vi "PersonnelFGV.vi"(7 "Actions":T1=enum."Read Personnel", 8 "error in (no error)":errorcluster, 9 "Data In":string, 10 "PUID":string) -> (0 "error out":errorcluster, 1 "Data Out":string)   [LabVIEW 2015]
uses:
  TypeDef/PersonnelActions.ctl
  TypeDef/PersonnelState.ctl
  LVClasses/Personnel/Personnel.lvclass
  LVClasses/Personnel/PersonnelType.ctl
  LVClasses/Personnel/Personnel.lvclass/Personnel.ctl
  LVClasses/Personnel/Read Name.vi
  LVClasses/Personnel/Read Role.vi
  LVClasses/Personnel/Read UniqueID.vi
  LVClasses/Personnel/Read Requests.vi
  LVClasses/Personnel/Write Requests.vi
  LVClasses/Personnel/Write Name.vi
  LVClasses/Personnel/Write Role.vi
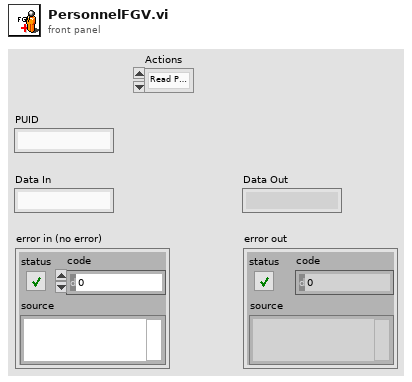
[diagram p1: front panel]
types:
  T1 = typedef "PersonnelActions.ctl" = enum16{"Init", "Read Personnel", "Add Personnel", "Remove Personnel", "Read Name", "Write Name", "Read Role", "Write Role", "Read Requests", "Add Requests", "Remove Requests", "Read PUIDs"}
  T2 = typedef "PersonnelState.ctl" = cluster{"Personnel":refnum<class "Personnel.lvclass">[]}
  T3 = typedef "Personnel.lvclass/PersonnelType.ctl" = enum16{"Nurse", "Doctor", "Cleanning", "Admin"}
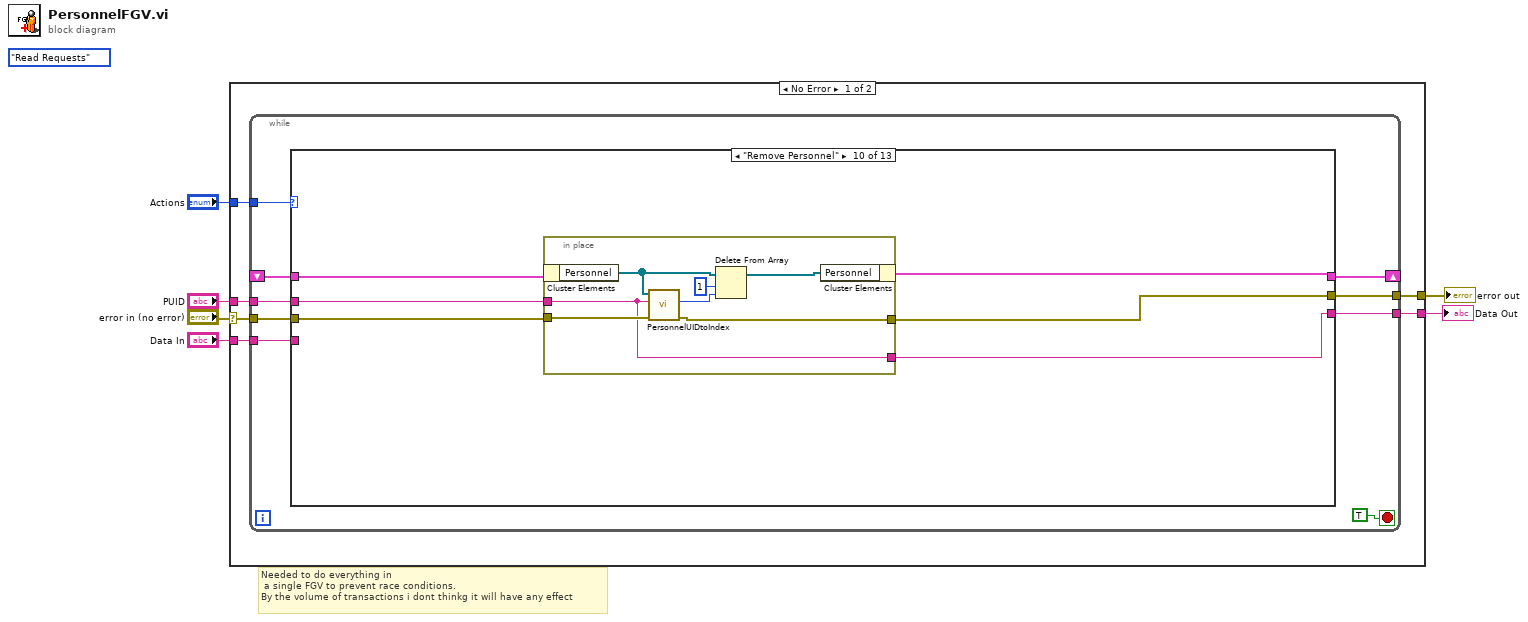
[diagram p0: block diagram]
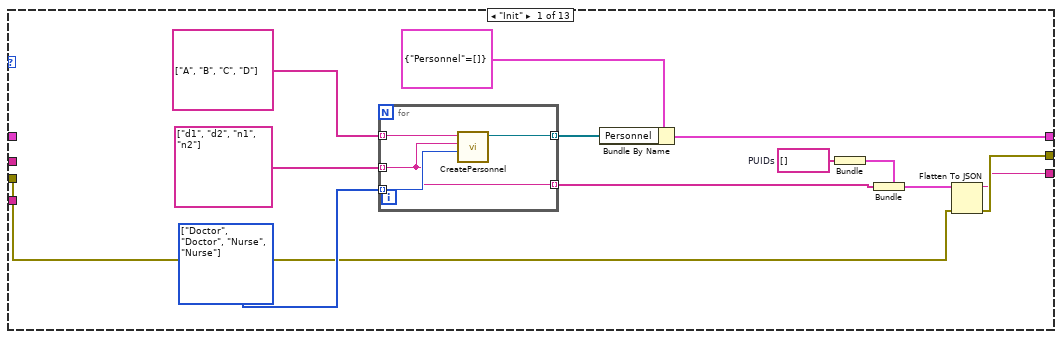
[diagram p2: hidden frame]
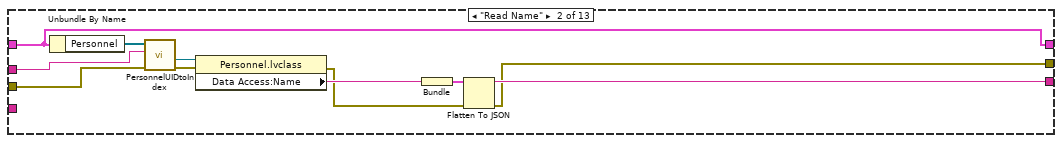
[diagram p3: hidden frame]
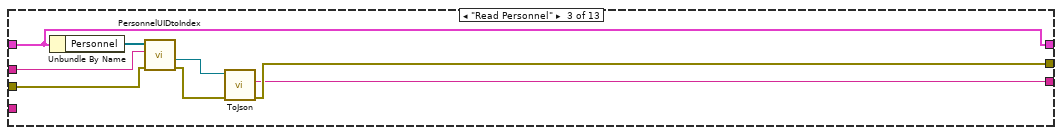
[diagram p4: hidden frame]
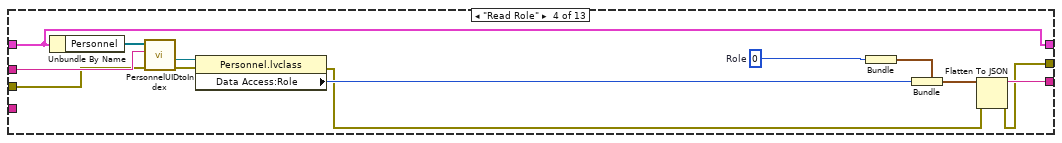
[diagram p5: hidden frame]
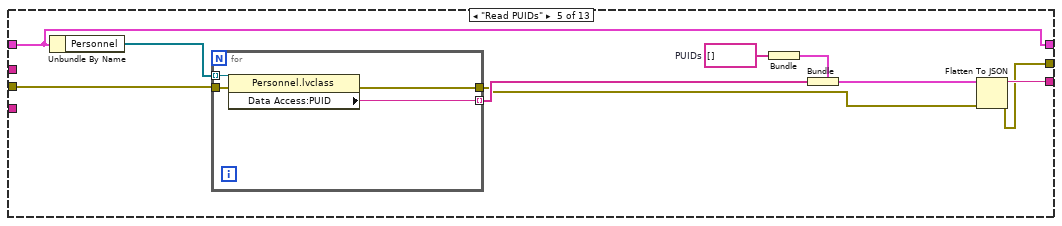
[diagram p6: hidden frame]
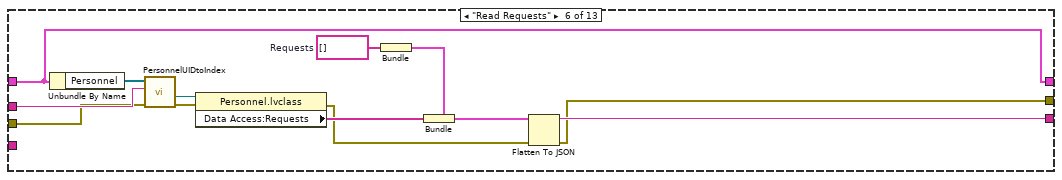
[diagram p7: hidden frame]
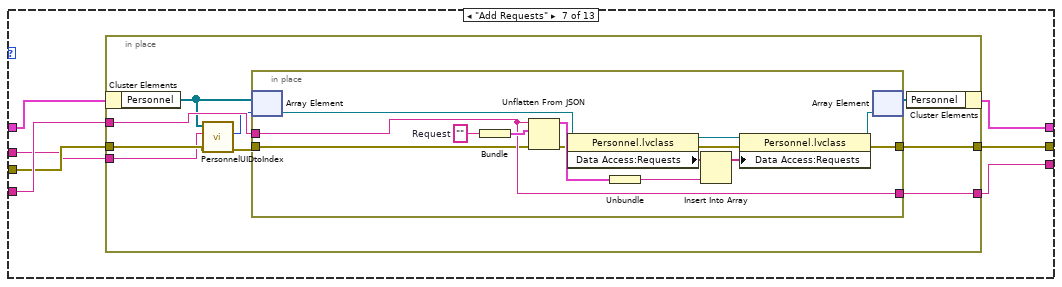
[diagram p8: hidden frame]
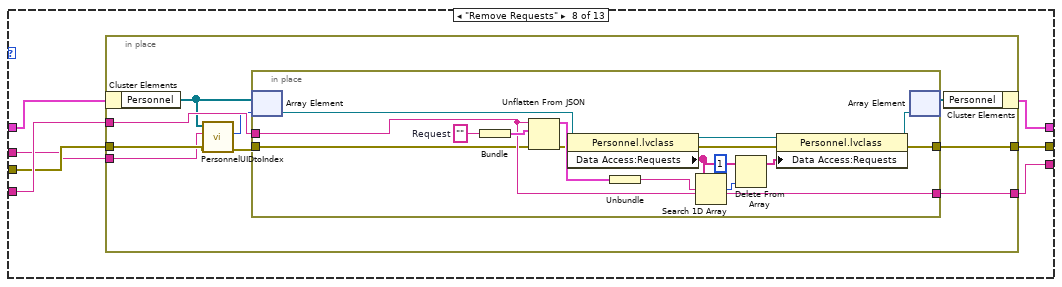
[diagram p9: hidden frame]
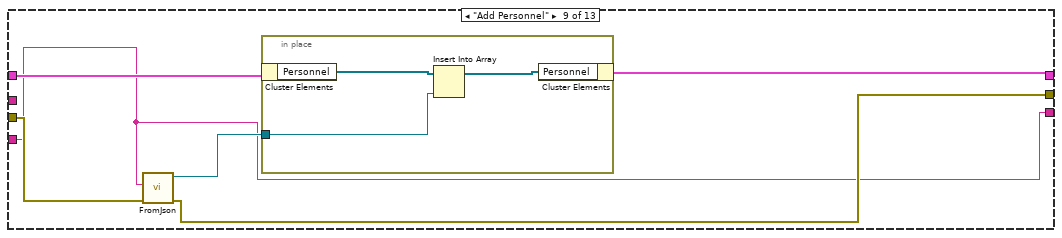
[diagram p10: hidden frame]
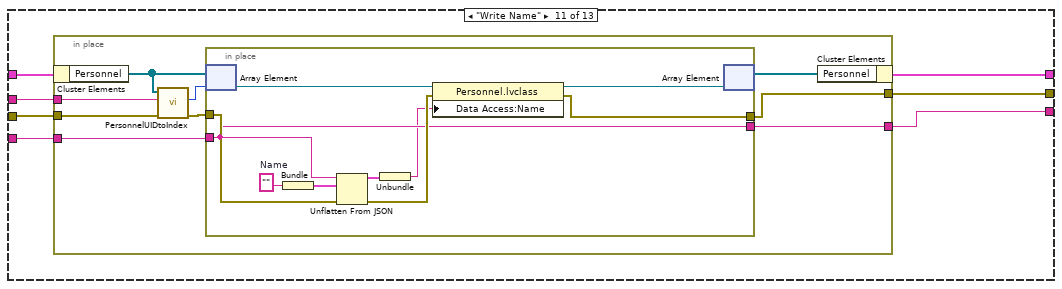
[diagram p11: hidden frame]
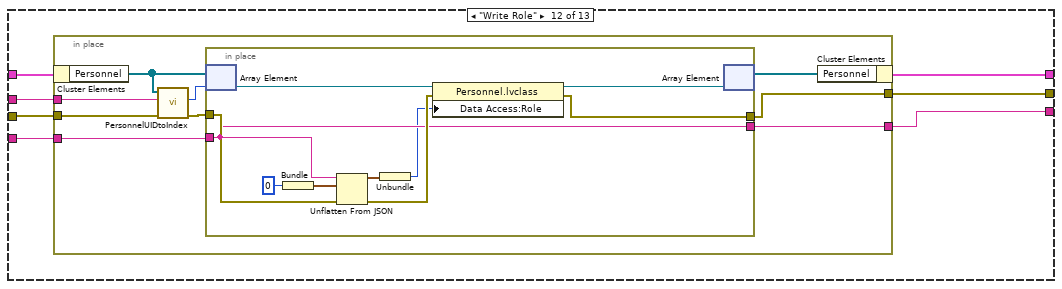
[diagram p12: hidden frame]
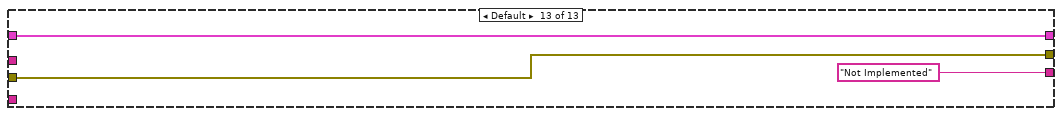
[diagram p13: hidden frame]
diagram:
  (unwired) PersonnelActions."Read Requests" ("Actions")
  # "Needed to do everything in\n a single FGV to prevent race conditions. \nBy the volume of transactions i dont thinkg it will have any effect"
  n1 = case shown="No Error" "error in (no error)" {
    selector: "error in (no error)" -> [w8 w237]
    tunnel: "Actions" -> [w12 _]
    tunnel: "PUID" -> [w11 _]
    tunnel: [w10 _] -> w4
    tunnel: "Data In" -> [w9 _]
    tunnel: [w7 w237] -> w1
    frame No Error {
      n2 = while {
        shift-right: [w19] -> _
        shift-left: _ -> [w18]
        tunnel: w12 -> [w20]
        tunnel: w11 -> [w17]
        tunnel: [w16] -> w10
        tunnel: w9 -> [w15]
        tunnel: w8 -> [w14]
        tunnel: [w13] -> w7
        stop <- TRUE ("stop") stop-if-true
        n3 = case shown="\"Remove Personnel\"" w20 {
          tunnel: [w34 w49 w57 w70 w80 w97 w99 w129 w161 w173 w187 w213 w236] -> w19
          tunnel: w18 -> [_ w49 w57 w70 w80 w97 w104 w134 w165 w174 w188 w214 w236]
          tunnel: w17 -> [_ w47 w55 w68 _ w95 w100 w130 _ w170 w184 w210 _]
          tunnel: [w22 w43 w50 w64 w79 w93 w98 w128 w160 w169 w182 w208 "Not Implemented" ("JSON string")] -> w16
          tunnel: w15 -> [_ _ _ _ _ _ w103 w133 w160 _ w183 w209 _]
          tunnel: w14 -> [w25 w42 w54 w61 w72 w88 w102 w132 w164 w172 w186 w212 w234]
          tunnel: [w26 w39 w51 w58 w78 w85 w101 w131 w163 w171 w185 w211 w234] -> w13
          frame "Init" {
            w27 = string[] []  # PUIDs
            w31 = T3[] [enum."Doctor", enum."Doctor", enum."Nurse", enum."Nurse"] items=["Nurse", "Doctor", "Cleanning", "Admin"]
            n4 = for {
              tunnel: [w38] -> w32 mode=indexing
              tunnel: w31 -> [w37] mode=indexing
              tunnel: string[] ["d1", "d2", "n1", "n2"] -> [w35] mode=indexing
              tunnel: string[] ["A", "B", "C", "D"] -> [w36] mode=indexing
              tunnel: [w35] -> w23 mode=indexing
              n5 = call "CreatePersonnel.vi"("Role"=w37, "UniqueID"=w35, "Name"=w36) -> ("output cluster"=w38:refnum<class "Personnel.lvclass">)  [unwired: 7 in, 1 out]
            }
            n6 = Bundle By Name(cluster=T2 {"Personnel"=[]}, "Personnel"=w32) -> (w34:T2)
            n7 = Bundle("PUIDs"=w27) -> (w28:cluster{"PUIDs":string[]})  [unwired: 1 in]
            n8 = Bundle(cluster=w28, "PUIDs"=w23) -> (w24:cluster{"PUIDs":string[]})
            n9 = Flatten To JSON(anything=w24, error in (no error)=w25) -> (JSON string=w22:string, 11:w26:errorcluster)  [unwired: 1 in]
          }
          frame "Read Name" {
            n10 = Unbundle By Name(w49) -> ("Personnel"=w48:refnum<class "Personnel.lvclass">[])
            n11 = call "PersonnelUIDtoIndex.vi"("error in (no error)"=w42, "PUID"=w47, "Personnel in"=w48) -> ("error out"=w41:errorcluster, "Personnel"=w46:refnum<class "Personnel.lvclass">)  [unwired: 5 in, 2 out]
            n12 = property class="Personnel.lvclass"(reference=w46, error in=w41) -> (error out=w40:errorcluster, "Data Access:Name"=w45:string)  [unwired: 1 out]
            n13 = Bundle("Data Access:Name"=w45) -> (w44:cluster{"Data Access:Name":string})  [unwired: 1 in]
            n14 = Flatten To JSON(anything=w44, error in (no error)=w40) -> (JSON string=w43:string, 11:w39:errorcluster)  [unwired: 1 in]
          }
          frame "Read Personnel" {
            n15 = Unbundle By Name(w57) -> ("Personnel"=w56:refnum<class "Personnel.lvclass">[])
            n16 = call "PersonnelUIDtoIndex.vi"("error in (no error)"=w54, "PUID"=w55, "Personnel in"=w56) -> ("error out"=w53:errorcluster, "Personnel"=w52:refnum<class "Personnel.lvclass">)  [unwired: 5 in, 2 out]
            n17 = call "ToJson.vi"("error in (no error)"=w53, "Personnel in"=w52) -> ("error out"=w51:errorcluster, "PersonnelJson"=w50:string)  [unwired: 7 in, 1 out]
          }
          frame "Read Role" {
            w63 = 0  # Role
            n18 = Unbundle By Name(w70) -> ("Personnel"=w69:refnum<class "Personnel.lvclass">[])
            n19 = call "PersonnelUIDtoIndex.vi"("error in (no error)"=w61, "PUID"=w68, "Personnel in"=w69) -> ("error out"=w60:errorcluster, "Personnel"=w67:refnum<class "Personnel.lvclass">)  [unwired: 5 in, 2 out]
            n20 = property class="Personnel.lvclass"(reference=w67, error in=w60) -> (error out=w59:errorcluster, "Data Access:Role"=w66:T3)  [unwired: 1 out]
            n21 = Bundle("Role"=w63) -> (w62:cluster{"Role":i32})  [unwired: 1 in]
            n22 = Bundle(cluster=w62, "Role"=w66) -> (w65:cluster{"Role":i32})
            n23 = Flatten To JSON(anything=w65, error in (no error)=w59) -> (JSON string=w64:string, 11:w58:errorcluster)  [unwired: 1 in]
          }
          frame "Read PUIDs" {
            w75 = string[] []  # PUIDs
            n24 = Unbundle By Name(w80) -> ("Personnel"=w77:refnum<class "Personnel.lvclass">[])
            n25 = for {
              tunnel: w77 -> [w84] mode=indexing
              tunnel: [w83] -> w73 mode=indexing
              tunnel: w72 -> [w82]
              tunnel: [w81] -> w71
              n26 = property class="Personnel.lvclass"(reference=w84, error in=w82) -> (error out=w81:errorcluster, "Data Access:PUID"=w83:string)  [unwired: 1 out]
            }
            n27 = Bundle("PUIDs"=w75) -> (w76:cluster{"PUIDs":string[]})  [unwired: 1 in]
            n28 = Bundle(cluster=w76, "PUIDs"=w73) -> (w74:cluster{"PUIDs":string[]})
            n29 = Flatten To JSON(anything=w74, error in (no error)=w71) -> (JSON string=w79:string, 11:w78:errorcluster)  [unwired: 1 in]
          }
          frame "Read Requests" {
            w91 = string[] []  # Requests
            n30 = Unbundle By Name(w97) -> ("Personnel"=w96:refnum<class "Personnel.lvclass">[])
            n31 = call "PersonnelUIDtoIndex.vi"("error in (no error)"=w88, "PUID"=w95, "Personnel in"=w96) -> ("error out"=w87:errorcluster, "Personnel"=w94:refnum<class "Personnel.lvclass">)  [unwired: 5 in, 2 out]
            n32 = property class="Personnel.lvclass"(reference=w94, error in=w87) -> (error out=w86:errorcluster, "Data Access:Requests"=w90:string[])  [unwired: 1 out]
            n33 = Bundle("Requests"=w91) -> (w92:cluster{"Requests":string[]})  [unwired: 1 in]
            n34 = Bundle(cluster=w92, "Requests"=w90) -> (w89:cluster{"Requests":string[]})
            n35 = Flatten To JSON(anything=w89, error in (no error)=w86) -> (JSON string=w93:string, 11:w85:errorcluster)  [unwired: 1 in]
          }
          frame "Add Requests" {
            n36 = in-place {
              in-place-border: [w111] -> w98
              in-place-border: w102 -> [w106]
              in-place-border: [w112] -> w101
              in-place-border: w103 -> [w110]
              in-place-border: w100 -> [w105]
              n37 = in-place-cluster #1(w104) -> ("Personnel"=w109:refnum<class "Personnel.lvclass">[])
              n38 = call "PersonnelUIDtoIndex.vi"("error in (no error)"=w106, "PUID"=w105, "Personnel in"=w109) -> ("error out"=w107:errorcluster, "Index"=w108:i32)  [unwired: 5 in, 2 out]
              n39 = in-place {
                in-place-border: w107 -> [w121]
                in-place-border: [w127] -> w112
                in-place-border: [w124] -> w111
                in-place-border: w110 -> [w124]
                w120 = ""  # Request
                n40 = in-place-array #2(w109, w108) -> (w122:refnum<class "Personnel.lvclass">)
                n41 = Bundle("Request"=w120) -> (w125:cluster{"Request":string})  [unwired: 1 in]
                n42 = Unflatten From JSON(JSON string=w124, type and defaults=w125, error in (no error)=w121) -> (value=w123:cluster{"Request":string}, error out=w118:errorcluster)  [unwired: 4 in]
                n43 = property class="Personnel.lvclass"(reference=w122, error in=w118) -> (reference out=w119:refnum<class "Personnel.lvclass">, error out=w117:errorcluster, "Data Access:Requests"=w116:string[])
                n44 = Unbundle(w123) -> ("Request"=w114:string)
                n45 = Insert Into Array(array=w116, new element=w114) -> (w115:string[])  [unwired: 1 in]
                n46 = property class="Personnel.lvclass"(reference=w119, error in=w117, "Data Access:Requests"=w115) -> (reference out=w126:refnum<class "Personnel.lvclass">, error out=w127:errorcluster)
                n47 = in-place-array #2(w126) -> (w113:refnum<class "Personnel.lvclass">[])  [unwired: 1 out]
              }
              n48 = in-place-cluster #1("Personnel"=w113) -> (w99:T2)
            }
          }
          frame "Remove Requests" {
            n49 = in-place {
              in-place-border: [w141] -> w128
              in-place-border: w132 -> [w136]
              in-place-border: [w142] -> w131
              in-place-border: w133 -> [w140]
              in-place-border: w130 -> [w135]
              n50 = in-place-cluster #3(w134) -> ("Personnel"=w139:refnum<class "Personnel.lvclass">[])
              n51 = call "PersonnelUIDtoIndex.vi"("error in (no error)"=w136, "PUID"=w135, "Personnel in"=w139) -> ("error out"=w137:errorcluster, "Index"=w138:i32)  [unwired: 5 in, 2 out]
              n52 = in-place {
                in-place-border: w137 -> [w153]
                in-place-border: [w159] -> w142
                in-place-border: [w156] -> w141
                in-place-border: w140 -> [w156]
                w152 = ""  # Request
                n53 = in-place-array #4(w139, w138) -> (w154:refnum<class "Personnel.lvclass">)
                n54 = Bundle("Request"=w152) -> (w157:cluster{"Request":string})  [unwired: 1 in]
                n55 = Unflatten From JSON(JSON string=w156, type and defaults=w157, error in (no error)=w153) -> (value=w155:cluster{"Request":string}, error out=w150:errorcluster)  [unwired: 4 in]
                n56 = property class="Personnel.lvclass"(reference=w154, error in=w150) -> (reference out=w151:refnum<class "Personnel.lvclass">, error out=w149:errorcluster, "Data Access:Requests"=w148:string[])
                n57 = Unbundle(w155) -> ("Request"=w144:string)
                n58 = Search 1D Array(1D array=w148, element=w144) -> (index of element=w146:i32)  [unwired: 1 in]
                n59 = Delete From Array(array=w148, length=1, index=w146) -> (array with subset deleted=w147:string[])  [unwired: 1 out]
                n60 = property class="Personnel.lvclass"(reference=w151, error in=w149, "Data Access:Requests"=w147) -> (reference out=w158:refnum<class "Personnel.lvclass">, error out=w159:errorcluster)
                n61 = in-place-array #4(w158) -> (w143:refnum<class "Personnel.lvclass">[])  [unwired: 1 out]
              }
              n62 = in-place-cluster #3("Personnel"=w143) -> (w129:T2)
            }
          }
          frame "Add Personnel" {
            n63 = call "FromJson.vi"("error in (no error)"=w164, "PersonnelJson"=w160) -> ("error out"=w163:errorcluster, "Personnel out"=w162:refnum<class "Personnel.lvclass">)  [unwired: 8 in]
            n64 = in-place {
              in-place-border: w162 -> [w166]
              n65 = in-place-cluster #5(w165) -> ("Personnel"=w168:refnum<class "Personnel.lvclass">[])
              n66 = Insert Into Array(array=w168, new element=w166) -> (w167:refnum<class "Personnel.lvclass">[])  [unwired: 1 in]
              n67 = in-place-cluster #5("Personnel"=w167) -> (w161:T2)
            }
          }
          frame "Remove Personnel" {
            n68 = in-place {
              in-place-border: w170 -> [w175]
              in-place-border: w172 -> [w180]
              in-place-border: [w176] -> w171
              in-place-border: [w175] -> w169
              n69 = in-place-cluster #6(w174) -> ("Personnel"=w179:refnum<class "Personnel.lvclass">[])
              n70 = call "PersonnelUIDtoIndex.vi"("error in (no error)"=w180, "PUID"=w175, "Personnel in"=w179) -> ("error out"=w176:errorcluster, "Index"=w177:i32)  [unwired: 5 in, 2 out]
              n71 = Delete From Array(array=w179, length=1, index=w177) -> (array with subset deleted=w181:refnum<class "Personnel.lvclass">[])  [unwired: 1 out]
              n72 = in-place-cluster #6("Personnel"=w181) -> (w173:T2)
            }
          }
          frame "Write Name" {
            n73 = in-place {
              in-place-border: w184 -> [w197]
              in-place-border: w186 -> [w196]
              in-place-border: [w190] -> w185
              in-place-border: w183 -> [w192]
              in-place-border: [w189] -> w182
              n74 = in-place-cluster #7(w188) -> ("Personnel"=w195:refnum<class "Personnel.lvclass">[])
              n75 = call "PersonnelUIDtoIndex.vi"("error in (no error)"=w196, "PUID"=w197, "Personnel in"=w195) -> ("error out"=w191:errorcluster, "Index"=w193:i32)  [unwired: 5 in, 2 out]
              n76 = in-place {
                in-place-border: w192 -> [w202]
                in-place-border: w191 -> [w205]
                in-place-border: [w203] -> w190
                in-place-border: [w202] -> w189
                w201 = ""  # Name
                n77 = in-place-array #8(w195, w193) -> (w207:refnum<class "Personnel.lvclass">)
                n78 = Bundle("Name"=w201) -> (w200:cluster{"Name":string})  [unwired: 1 in]
                n79 = Unflatten From JSON(JSON string=w202, type and defaults=w200, error in (no error)=w205) -> (value=w199:cluster{"Name":string}, error out=w204:errorcluster)  [unwired: 4 in]
                n80 = Unbundle(w199) -> ("Name"=w198:string)
                n81 = property class="Personnel.lvclass"(reference=w207, error in=w204, "Data Access:Name"=w198) -> (reference out=w206:refnum<class "Personnel.lvclass">, error out=w203:errorcluster)
                n82 = in-place-array #8(w206) -> (w194:refnum<class "Personnel.lvclass">[])  [unwired: 1 out]
              }
              n83 = in-place-cluster #7("Personnel"=w194) -> (w187:T2)
            }
          }
          frame "Write Role" {
            n84 = in-place {
              in-place-border: w210 -> [w223]
              in-place-border: w212 -> [w222]
              in-place-border: [w216] -> w211
              in-place-border: w209 -> [w218]
              in-place-border: [w215] -> w208
              n85 = in-place-cluster #9(w214) -> ("Personnel"=w221:refnum<class "Personnel.lvclass">[])
              n86 = call "PersonnelUIDtoIndex.vi"("error in (no error)"=w222, "PUID"=w223, "Personnel in"=w221) -> ("error out"=w217:errorcluster, "Index"=w219:i32)  [unwired: 5 in, 2 out]
              n87 = in-place {
                in-place-border: w218 -> [w228]
                in-place-border: w217 -> [w231]
                in-place-border: [w229] -> w216
                in-place-border: [w228] -> w215
                n88 = in-place-array #10(w221, w219) -> (w233:refnum<class "Personnel.lvclass">)
                n89 = Bundle("Role"=0) -> (w227:cluster{"Role":i32})  [unwired: 1 in]
                n90 = Unflatten From JSON(JSON string=w228, type and defaults=w227, error in (no error)=w231) -> (value=w226:cluster{"Role":i32}, error out=w230:errorcluster)  [unwired: 4 in]
                n91 = Unbundle(w226) -> ("Role"=w225:i32)
                n92 = property class="Personnel.lvclass"(reference=w233, error in=w230, "Data Access:Role"=w225) -> (reference out=w232:refnum<class "Personnel.lvclass">, error out=w229:errorcluster)
                n93 = in-place-array #10(w232) -> (w220:refnum<class "Personnel.lvclass">[])  [unwired: 1 out]
              }
              n94 = in-place-cluster #9("Personnel"=w220) -> (w213:T2)
            }
          }
          frame Default {
          }
        }
      }
    }
    frame Error {
    }
  }
  "Data Out" <- w4
  "error out" <- w1
